vi "Calculate Normals.vi"(9 "Color Binding Mode":T1(ring), 10 "Vertex Array":cluster{"X":sgl, "Y":sgl, "Z":sgl}[](array[cluster]), 11 "Draw Mode":T2(ring)) -> (3 "Normal Array":cluster{"X":sgl, "Y":sgl, "Z":sgl}[](array[cluster]))   [LabVIEW 2023]
doc: "Calculates Normal values of the vertices."
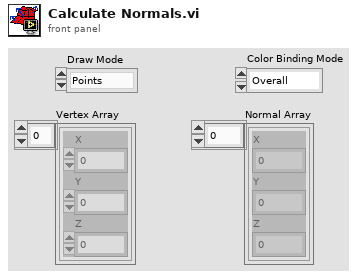
[diagram p1: front panel]
types:
  T1 = enum16{"Overall", "Per Primitive", "Per Vertex", "Binding Off"}
  T2 = enum16{"Points", "Lines", "Line Strip", "Line Loop", "Triangles", "Triangle Strip", "Triangle Fan", "Quads", "Quad Strip", "Polygon"}
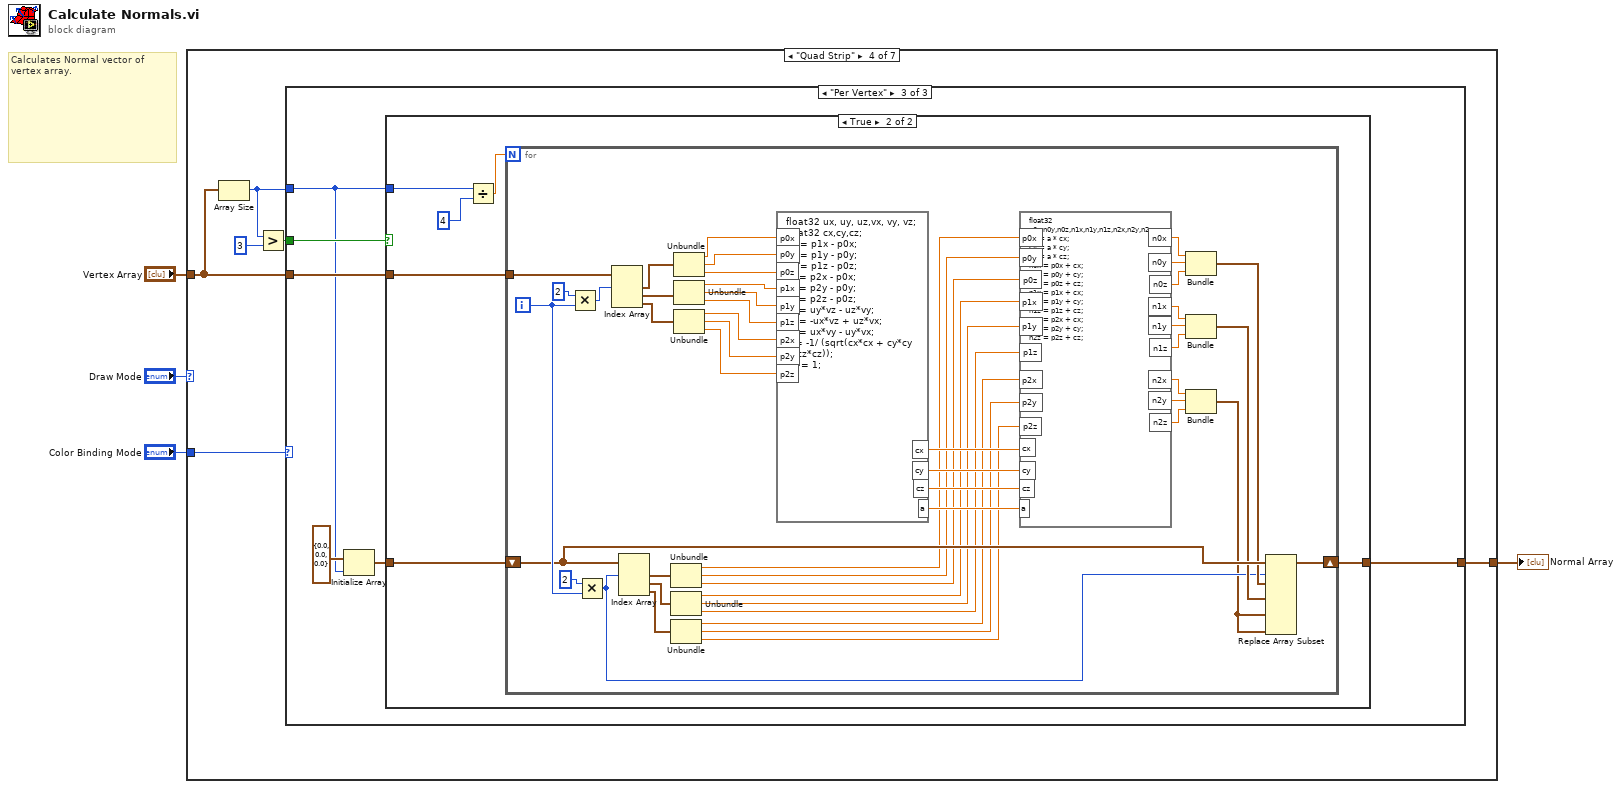
[diagram p0: block diagram]
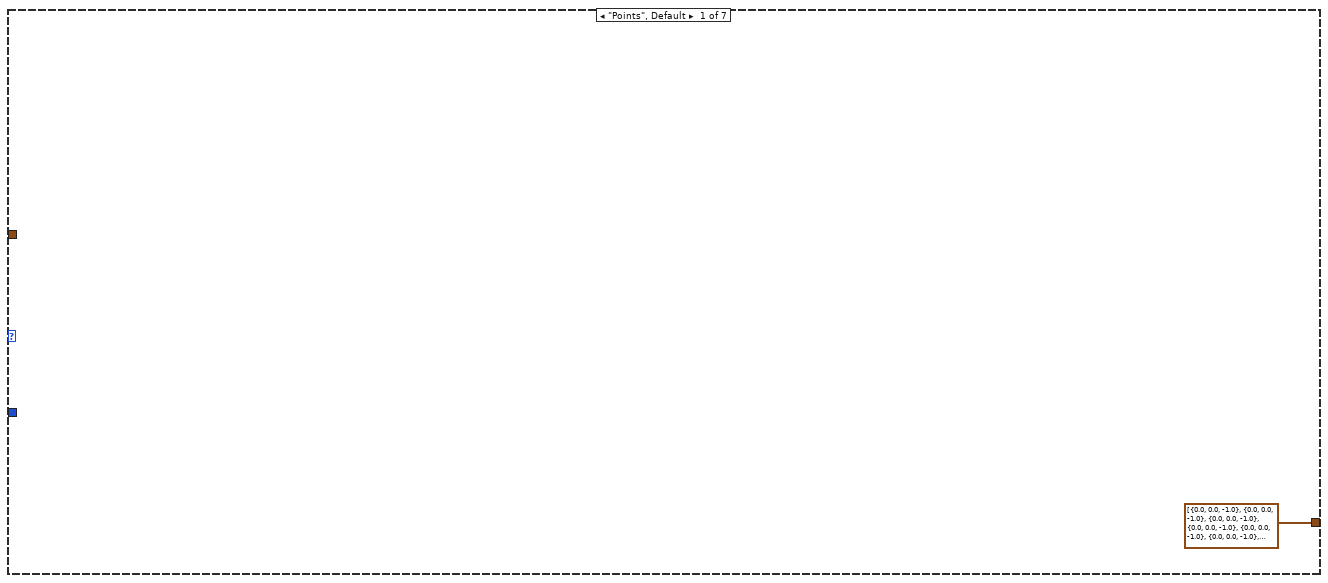
[diagram p2: hidden frame]
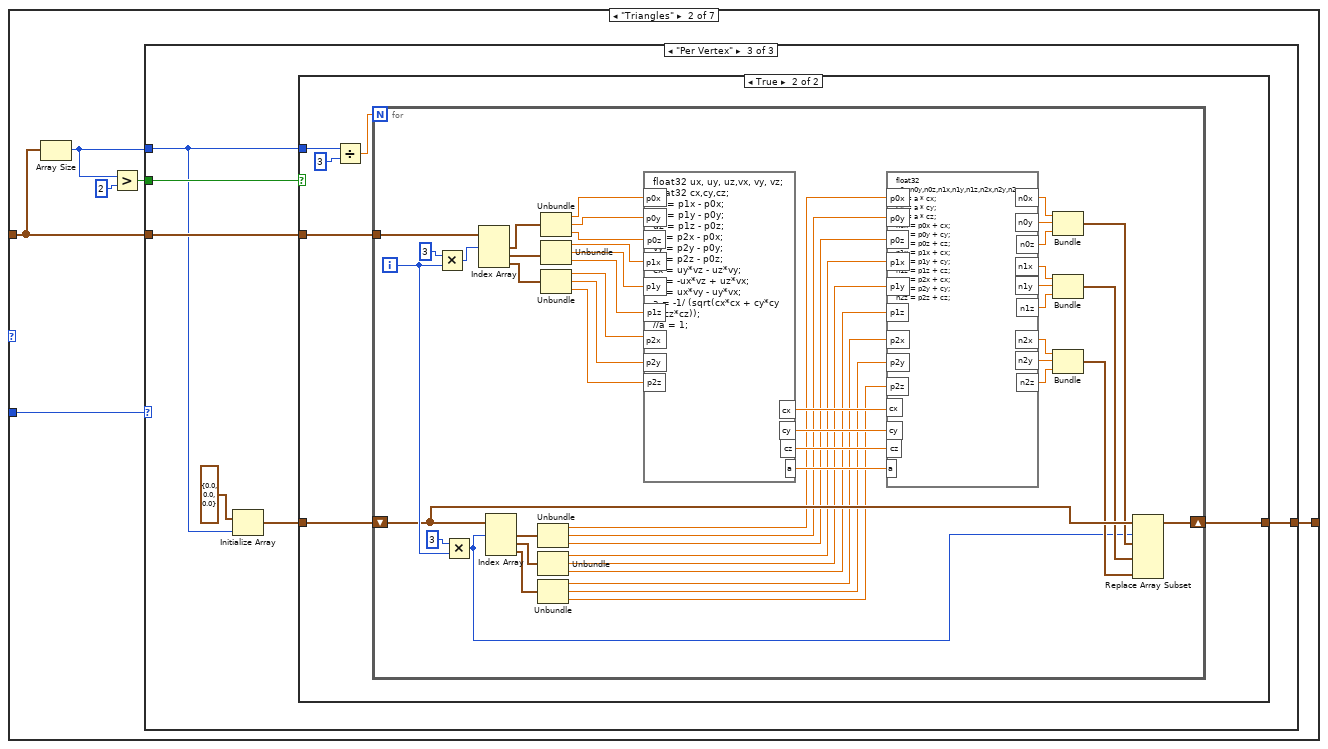
[diagram p3: hidden frame]
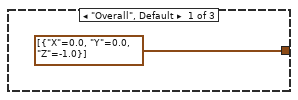
[diagram p4: hidden frame]
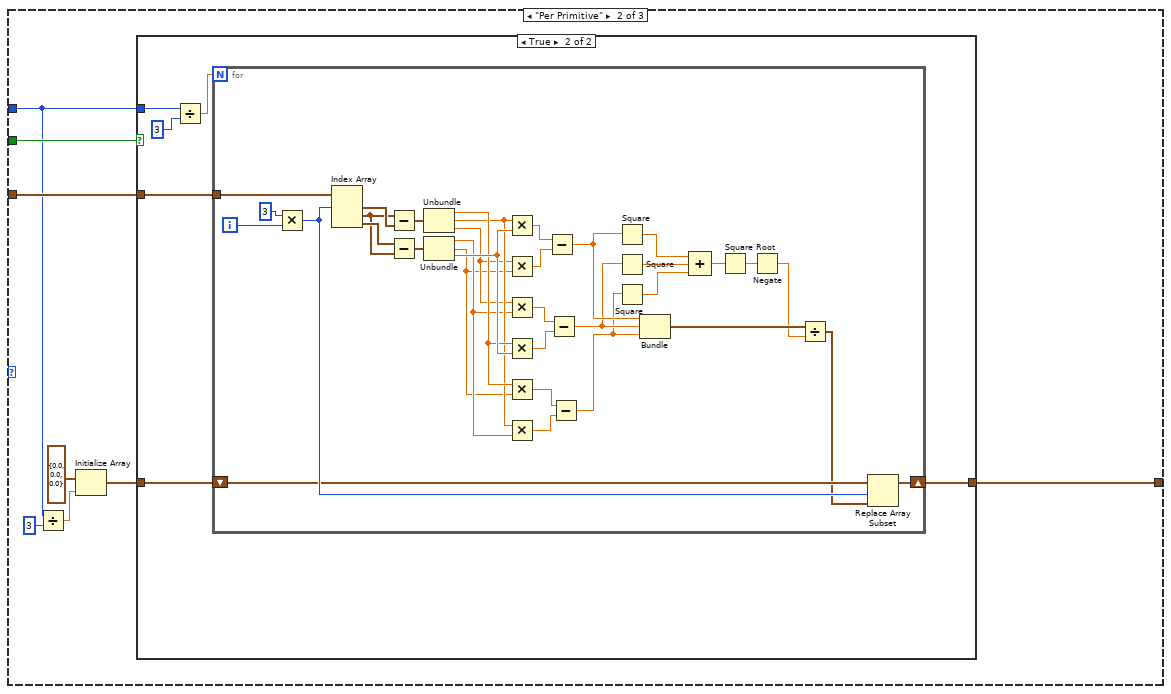
[diagram p5: hidden frame]
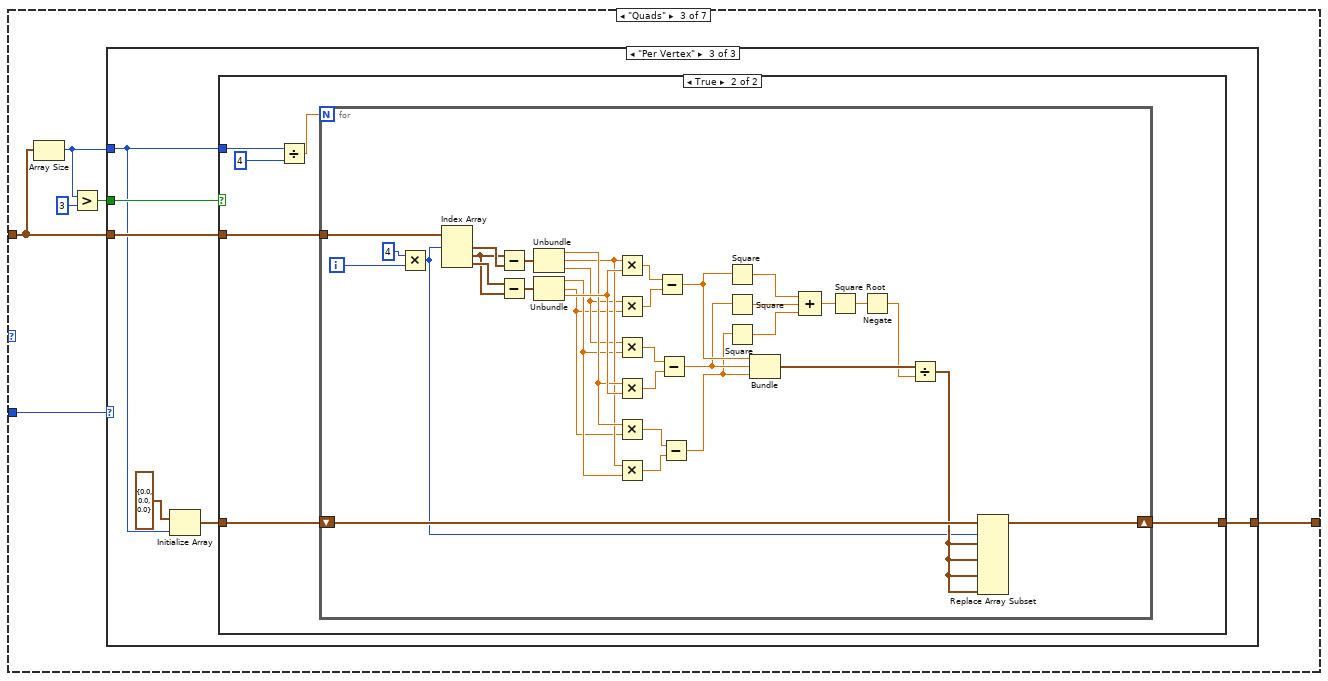
[diagram p8: hidden frame]
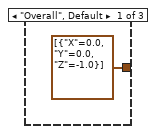
[diagram p9: hidden frame]
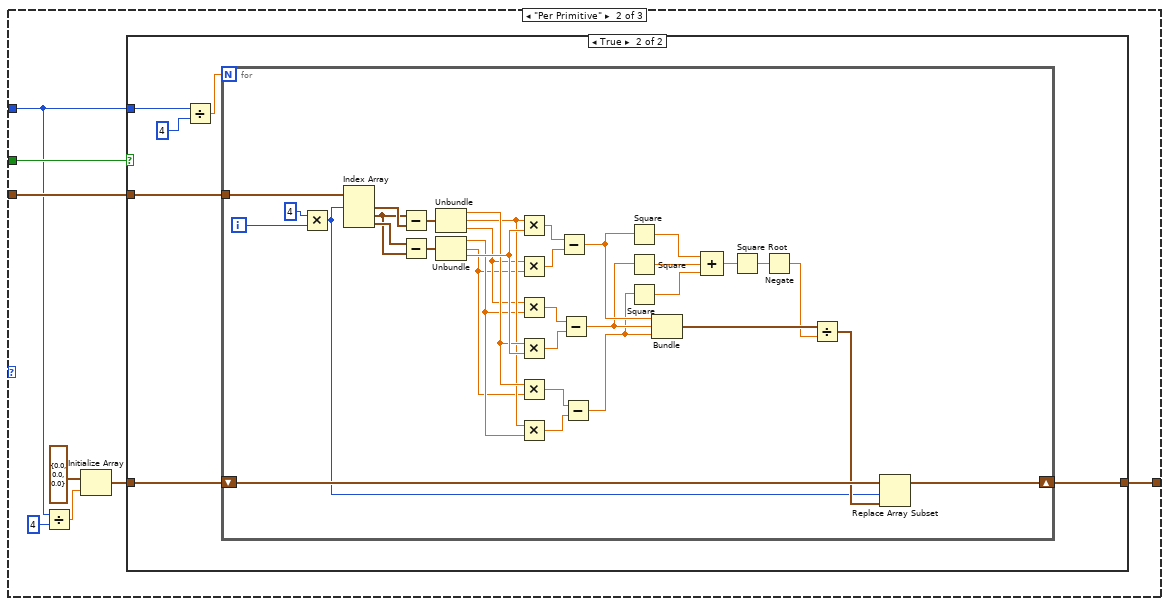
[diagram p10: hidden frame]
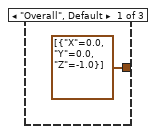
[diagram p13: hidden frame]
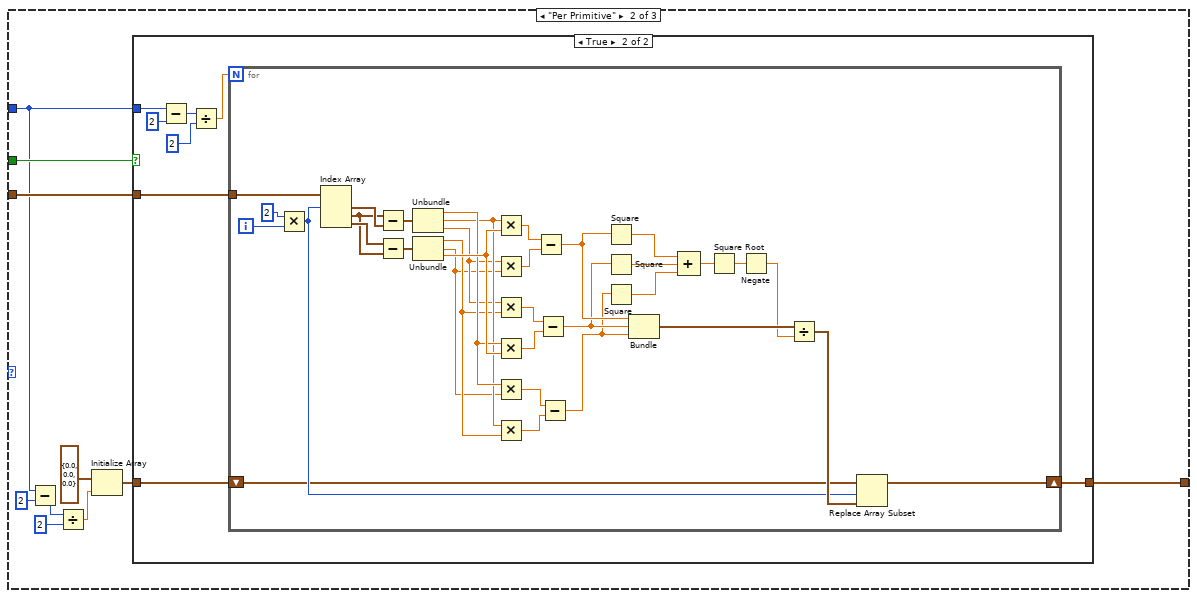
[diagram p14: hidden frame]
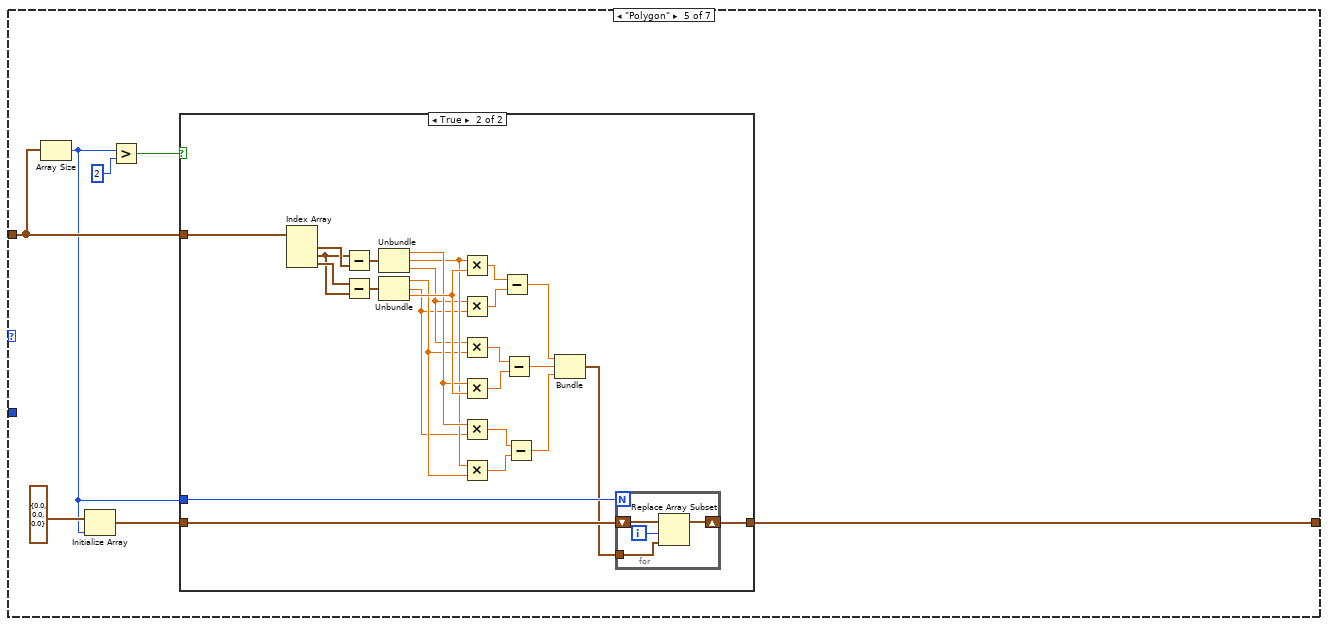
[diagram p17: hidden frame]
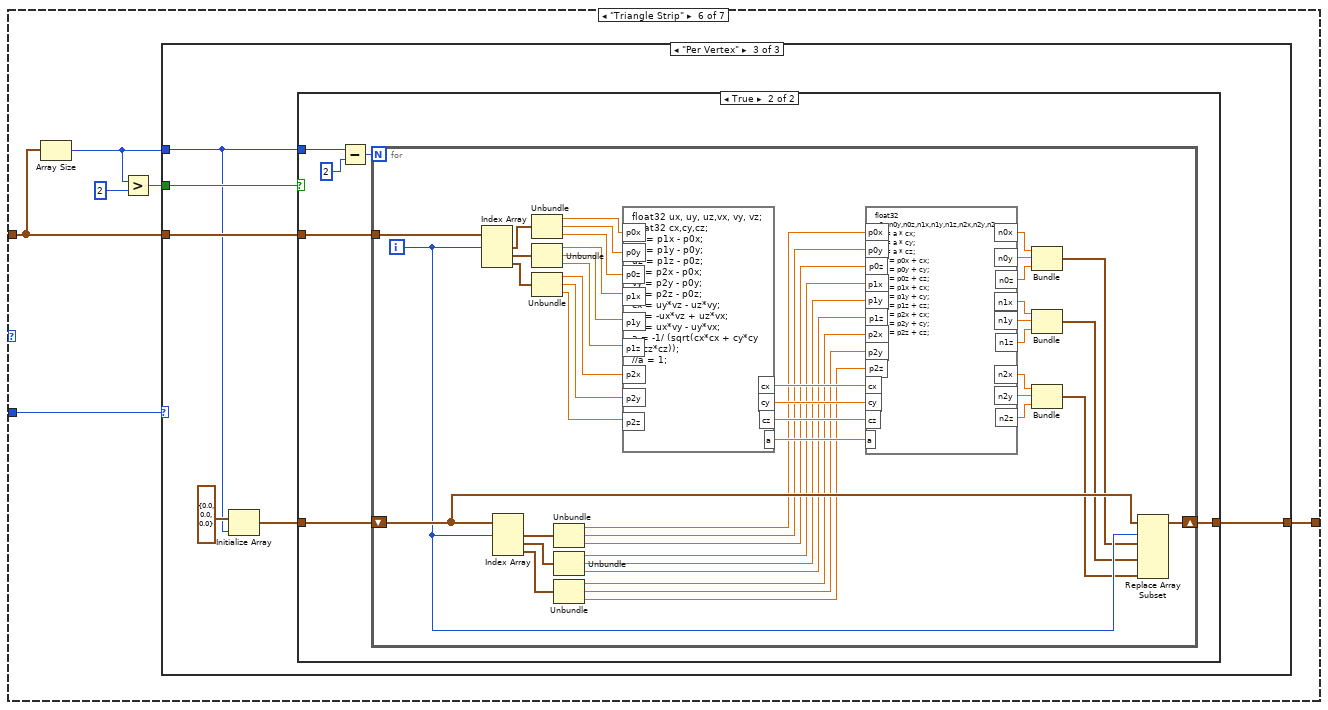
[diagram p19: hidden frame]
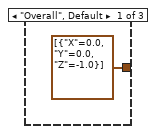
[diagram p20: hidden frame]
diagram:
  # "Calculates Normal vector of  vertex array."
  n1 = case shown="\"Quad Strip\"" "Draw Mode" {
    tunnel: "Vertex Array" -> [_ w11 w126 w227 w347 w382 w490]
    tunnel: [cluster{"X":sgl, "Y":sgl, "Z":sgl}[] [{"X"=0.0, "Y"=0.0, "Z"=-1.0}, {"X"=0.0, "Y"=0.0, "Z"=-1.0}, {"X"=0.0, "Y"=0.0, "Z"=-1.0}, {"X"=0.0, "Y"=0.0, "Z"=-1.0}, {"X"=0.0, "Y"=0.0, "Z"=-1.0}, {"X"=0.0, "Y"=0.0, "Z"=-1.0}, {"X"=0.0, "Y"=0.0, "Z"=-1.0}, {"X"=0.0, "Y"=0.0, "Z"=-1.0}, {"X"=0.0, "Y"=0.0, "Z"=-1.0}, {"X"=0.0, "Y"=0.0, "Z"=-1.0}] w10 w125 w226 w341 w381 w489] -> w2
    tunnel: "Color Binding Mode" -> [_ w7 w122 w222 _ w377 w485]
    frame "Points", Default {
    }
    frame "Triangles" {
      n2 = Array Size(array=w11) -> (size(s)=w6:i32)
      n3 = Greater?(x=w6, y=2) -> (0:w8:bool)
      n4 = case shown="\"Per Vertex\"" w7 {
        tunnel: w11 -> [_ w20 w66]
        tunnel: [cluster{"X":sgl, "Y":sgl, "Z":sgl}[] [{"X"=0.0, "Y"=0.0, "Z"=-1.0}] w19 w65] -> w10
        tunnel: w6 -> [_ w13 w61]
        tunnel: w8 -> [_ w18 w64]
        frame "Overall", Default {
        }
        frame "Per Primitive" {
          n5 = Divide(x=w13, y=3) -> (x/y=w15:dbl)
          n6 = Initialize Array(cluster{"X":sgl, "Y":sgl, "Z":sgl} {"X"=0.0, "Y"=0.0, "Z"=0.0} ("element"), w15) -> (w14:cluster{"X":sgl, "Y":sgl, "Z":sgl}[])
          n7 = case shown="True" w18 {
            tunnel: w20 -> [_ w26]
            tunnel: w14 -> [_ w23]
            tunnel: [_ w22] -> w19
            tunnel: w13 -> [_ w21]
            frame False {
            }
            frame True {
              n8 = Divide(x=w21, y=3) -> (x/y=w24:dbl)
              n9 = for {
                N: w24 -> [_]
                tunnel: w26 -> [w33]
                shift-right: [w29] -> w22
                shift-left: w23 -> [w31]
                i -> [w60]
                n10 = Multiply(x=3, y=w60) -> (x*y=w32:i32)
                n11 = Index Array(array=w33, index #1=w32) -> (element #1=w57:cluster{"X":sgl, "Y":sgl, "Z":sgl}, element #2=w56:cluster{"X":sgl, "Y":sgl, "Z":sgl}, element #3=w58:cluster{"X":sgl, "Y":sgl, "Z":sgl})  [unwired: 2 in]
                n12 = Subtract(x=w56, y=w57) -> (x-y=w54:cluster{"X":sgl, "Y":sgl, "Z":sgl})
                n13 = Subtract(x=w58, y=w56) -> (x-y=w55:cluster{"X":sgl, "Y":sgl, "Z":sgl})
                n14 = Unbundle(w54) -> ("X"=w52:sgl, "Y"=w51:sgl, "Z"=w50:sgl)
                n15 = Unbundle(w55) -> ("X"=w49:sgl, "Y"=w48:sgl, "Z"=w53:sgl)
                n16 = Multiply(x=w51, y=w53) -> (x*y=w47:sgl)
                n17 = Multiply(x=w50, y=w48) -> (x*y=w46:sgl)
                n18 = Multiply(x=w50, y=w49) -> (x*y=w44:sgl)
                n19 = Multiply(x=w52, y=w53) -> (x*y=w45:sgl)
                n20 = Multiply(x=w52, y=w48) -> (x*y=w42:sgl)
                n21 = Multiply(x=w51, y=w49) -> (x*y=w43:sgl)
                n22 = Subtract(x=w47, y=w46) -> (x-y=w39:sgl)
                n23 = Subtract(x=w44, y=w45) -> (x-y=w38:sgl)
                n24 = Subtract(x=w42, y=w43) -> (x-y=w37:sgl)
                n25 = Square(x=w39) -> (x^2=w28:sgl)
                n26 = Square(x=w38) -> (x^2=w27:sgl)
                n27 = Square(x=w37) -> (x^2=w41:sgl)
                n28 = Bundle(w39, w38, w37) -> (w36:cluster{sgl, sgl, sgl})  [unwired: 1 in]
                n29 = Compound Arithmetic op=ADD(w28, w27, w41) -> (w40:sgl)
                n30 = Square Root(x=w40) -> (sqrt(x)=w35:sgl)
                n31 = Negate(x=w35) -> (-x=w34:sgl)
                n32 = Divide(x=w36, y=w34) -> (x/y=w30:cluster{sgl, sgl, sgl})
                n33 = Replace Array Subset(array=w31, new element=w30, index=w32) -> (w29:cluster{"X":sgl, "Y":sgl, "Z":sgl}[])
              }
            }
          }
        }
        frame "Per Vertex" {
          n34 = Initialize Array(cluster{"X":sgl, "Y":sgl, "Z":sgl} {"X"=0.0, "Y"=0.0, "Z"=0.0} ("element"), w61) -> (w62:cluster{"X":sgl, "Y":sgl, "Z":sgl}[])
          n35 = case shown="True" w64 {
            tunnel: w66 -> [_ w72]
            tunnel: w62 -> [_ w69]
            tunnel: [_ w68] -> w65
            tunnel: w61 -> [_ w67]
            frame False {
            }
            frame True {
              n36 = Divide(x=w67, y=3) -> (x/y=w70:dbl)
              n37 = for {
                N: w70 -> [_]
                tunnel: w72 -> [w120]
                shift-right: [w117] -> w68
                shift-left: w69 -> [w118]
                i -> [w119]
                n38 = Multiply(x=3, y=w119) -> (x*y=w115:i32)
                n39 = Multiply(x=3, y=w119) -> (x*y=w73:i32)
                n40 = Index Array(array=w120, index #1=w115) -> (element #1=w98:cluster{"X":sgl, "Y":sgl, "Z":sgl}, element #2=w99:cluster{"X":sgl, "Y":sgl, "Z":sgl}, element #3=w100:cluster{"X":sgl, "Y":sgl, "Z":sgl})  [unwired: 2 in]
                n41 = Index Array(array=w118, index #1=w73) -> (element #1=w88:cluster{"X":sgl, "Y":sgl, "Z":sgl}, element #2=w87:cluster{"X":sgl, "Y":sgl, "Z":sgl}, element #3=w86:cluster{"X":sgl, "Y":sgl, "Z":sgl})  [unwired: 2 in]
                n42 = Unbundle(w88) -> ("X"=w85:sgl, "Y"=w84:sgl, "Z"=w83:sgl)
                n43 = Unbundle(w87) -> ("X"=w82:sgl, "Y"=w81:sgl, "Z"=w80:sgl)
                n44 = Unbundle(w86) -> ("X"=w79:sgl, "Y"=w78:sgl, "Z"=w77:sgl)
                n45 = Unbundle(w98) -> ("X"=w97:sgl, "Y"=w96:sgl, "Z"=w95:sgl)
                n46 = Unbundle(w99) -> ("X"=w94:sgl, "Y"=w93:sgl, "Z"=w92:sgl)
                n47 = Unbundle(w100) -> ("X"=w91:sgl, "Y"=w90:sgl, "Z"=w89:sgl)
                n48 = formula code="float32 ux, uy, uz,vx, vy, vz; \nfloat32 cx,cy,cz; \nux = p1x - p0x; \nuy = p1y - p0y; \nuz = p1z - p0z; \nvx = p2x - p0x; \nvy = p2y - p0y; \nvz = p2z - p0z; \ncx = uy*vz - uz*vy;\ncy = -ux*vz + uz*vx;\ncz = ux*vy - uy*vx;\na = -1/ (sqrt(cx*cx + cy*cy + cz*cz));\n//a = 1;"("p0x"=w97, "p0y"=w96, "p0z"=w95, "p1x"=w94, "p1y"=w93, "p1z"=w92, "p2x"=w91, "p2y"=w90, "p2z"=w89) -> ("cx"=w104:sgl, "cy"=w103:sgl, "cz"=w102:sgl, "a"=w105:dbl)
                n49 = formula code="float32 n0x,n0y,n0z,n1x,n1y,n1z,n2x,n2y,n2z;\ncx = a * cx; \ncy = a * cy; \ncz = a * cz; \nn0x = p0x + cx; \nn0y = p0y + cy;\nn0z = p0z + cz;\nn1x = p1x + cx; \nn1y = p1y + cy;\nn1z = p1z + cz;\nn2x = p2x + cx; \nn2y = p2y + cy;\nn2z = p2z + cz;"("p0x"=w85, "p0y"=w84, "p0z"=w83, "p1x"=w82, "p1y"=w81, "p1z"=w80, "p2x"=w79, "p2y"=w78, "p2z"=w77, "cx"=w104, "cy"=w103, "cz"=w102, "a"=w105) -> ("n0x"=w114:sgl, "n0y"=w113:sgl, "n0z"=w112:sgl, "n1x"=w111:sgl, "n1y"=w110:sgl, "n1z"=w109:sgl, "n2x"=w108:sgl, "n2y"=w107:sgl, "n2z"=w106:sgl)
                n50 = Bundle(w114, w113, w112) -> (w76:cluster{sgl, sgl, sgl})  [unwired: 1 in]
                n51 = Bundle(w111, w110, w109) -> (w75:cluster{sgl, sgl, sgl})  [unwired: 1 in]
                n52 = Bundle(w108, w107, w106) -> (w74:cluster{sgl, sgl, sgl})  [unwired: 1 in]
                n53 = Replace Array Subset(array=w118, new element #1=w76, index #1=w73, new element #2=w75, new element #3=w74) -> (w117:cluster{"X":sgl, "Y":sgl, "Z":sgl}[])  [unwired: 2 in]
              }
            }
          }
        }
      }
    }
    frame "Quads" {
      n54 = Array Size(array=w126) -> (size(s)=w121:i32)
      n55 = Greater?(x=w121, y=3) -> (0:w123:bool)
      n56 = case shown="\"Per Vertex\"" w122 {
        tunnel: w126 -> [_ w135 w181]
        tunnel: [cluster{"X":sgl, "Y":sgl, "Z":sgl}[] [{"X"=0.0, "Y"=0.0, "Z"=-1.0}] w134 w180] -> w125
        tunnel: w121 -> [_ w128 w177]
        tunnel: w123 -> [_ w133 w179]
        frame "Overall", Default {
        }
        frame "Per Primitive" {
          n57 = Divide(x=w128, y=4) -> (x/y=w130:dbl)
          n58 = Initialize Array(cluster{"X":sgl, "Y":sgl, "Z":sgl} {"X"=0.0, "Y"=0.0, "Z"=0.0} ("element"), w130) -> (w129:cluster{"X":sgl, "Y":sgl, "Z":sgl}[])
          n59 = case shown="True" w133 {
            tunnel: w135 -> [_ w139]
            tunnel: w129 -> [_ w137]
            tunnel: [_ w136] -> w134
            tunnel: w128 -> [_ w140]
            frame False {
            }
            frame True {
              n60 = Divide(x=w140, y=4) -> (x/y=w138:dbl)
              n61 = for {
                N: w138 -> [_]
                tunnel: w139 -> [w175]
                shift-right: [w172] -> w136
                shift-left: w137 -> [w173]
                i -> [w174]
                n62 = Multiply(x=4, y=w174) -> (x*y=w145:i32)
                n63 = Index Array(array=w175, index #1=w145) -> (element #1=w169:cluster{"X":sgl, "Y":sgl, "Z":sgl}, element #2=w168:cluster{"X":sgl, "Y":sgl, "Z":sgl}, element #3=w170:cluster{"X":sgl, "Y":sgl, "Z":sgl})  [unwired: 2 in]
                n64 = Subtract(x=w168, y=w169) -> (x-y=w166:cluster{"X":sgl, "Y":sgl, "Z":sgl})
                n65 = Subtract(x=w170, y=w168) -> (x-y=w167:cluster{"X":sgl, "Y":sgl, "Z":sgl})
                n66 = Unbundle(w166) -> ("X"=w164:sgl, "Y"=w163:sgl, "Z"=w162:sgl)
                n67 = Unbundle(w167) -> ("X"=w161:sgl, "Y"=w160:sgl, "Z"=w165:sgl)
                n68 = Multiply(x=w163, y=w165) -> (x*y=w159:sgl)
                n69 = Multiply(x=w162, y=w160) -> (x*y=w158:sgl)
                n70 = Multiply(x=w162, y=w161) -> (x*y=w156:sgl)
                n71 = Multiply(x=w164, y=w165) -> (x*y=w157:sgl)
                n72 = Multiply(x=w164, y=w160) -> (x*y=w154:sgl)
                n73 = Multiply(x=w163, y=w161) -> (x*y=w155:sgl)
                n74 = Subtract(x=w159, y=w158) -> (x-y=w151:sgl)
                n75 = Subtract(x=w156, y=w157) -> (x-y=w150:sgl)
                n76 = Subtract(x=w154, y=w155) -> (x-y=w149:sgl)
                n77 = Square(x=w151) -> (x^2=w143:sgl)
                n78 = Square(x=w150) -> (x^2=w142:sgl)
                n79 = Square(x=w149) -> (x^2=w153:sgl)
                n80 = Bundle(w151, w150, w149) -> (w148:cluster{sgl, sgl, sgl})  [unwired: 1 in]
                n81 = Compound Arithmetic op=ADD(w143, w142, w153) -> (w152:sgl)
                n82 = Square Root(x=w152) -> (sqrt(x)=w147:sgl)
                n83 = Negate(x=w147) -> (-x=w144:sgl)
                n84 = Divide(x=w148, y=w144) -> (x/y=w146:cluster{sgl, sgl, sgl})
                n85 = Replace Array Subset(array=w173, new element=w146, index=w145) -> (w172:cluster{"X":sgl, "Y":sgl, "Z":sgl}[])
              }
            }
          }
        }
        frame "Per Vertex" {
          n86 = Initialize Array(cluster{"X":sgl, "Y":sgl, "Z":sgl} {"X"=0.0, "Y"=0.0, "Z"=0.0} ("element"), w177) -> (w176:cluster{"X":sgl, "Y":sgl, "Z":sgl}[])
          n87 = case shown="True" w179 {
            tunnel: w181 -> [_ w185]
            tunnel: w176 -> [_ w183]
            tunnel: [_ w182] -> w180
            tunnel: w177 -> [_ w186]
            frame False {
            }
            frame True {
              n88 = Divide(x=w186, y=4) -> (x/y=w184:dbl)
              n89 = for {
                N: w184 -> [_]
                tunnel: w185 -> [w221]
                shift-right: [w218] -> w182
                shift-left: w183 -> [w219]
                i -> [w220]
                n90 = Multiply(x=4, y=w220) -> (x*y=w191:i32)
                n91 = Index Array(array=w221, index #1=w191) -> (element #1=w215:cluster{"X":sgl, "Y":sgl, "Z":sgl}, element #2=w214:cluster{"X":sgl, "Y":sgl, "Z":sgl}, element #3=w216:cluster{"X":sgl, "Y":sgl, "Z":sgl})  [unwired: 2 in]
                n92 = Subtract(x=w214, y=w215) -> (x-y=w212:cluster{"X":sgl, "Y":sgl, "Z":sgl})
                n93 = Subtract(x=w216, y=w214) -> (x-y=w213:cluster{"X":sgl, "Y":sgl, "Z":sgl})
                n94 = Unbundle(w212) -> ("X"=w210:sgl, "Y"=w209:sgl, "Z"=w208:sgl)
                n95 = Unbundle(w213) -> ("X"=w207:sgl, "Y"=w206:sgl, "Z"=w211:sgl)
                n96 = Multiply(x=w209, y=w211) -> (x*y=w205:sgl)
                n97 = Multiply(x=w208, y=w206) -> (x*y=w204:sgl)
                n98 = Multiply(x=w208, y=w207) -> (x*y=w202:sgl)
                n99 = Multiply(x=w210, y=w211) -> (x*y=w203:sgl)
                n100 = Multiply(x=w210, y=w206) -> (x*y=w200:sgl)
                n101 = Multiply(x=w209, y=w207) -> (x*y=w201:sgl)
                n102 = Subtract(x=w205, y=w204) -> (x-y=w197:sgl)
                n103 = Subtract(x=w202, y=w203) -> (x-y=w196:sgl)
                n104 = Subtract(x=w200, y=w201) -> (x-y=w195:sgl)
                n105 = Square(x=w197) -> (x^2=w189:sgl)
                n106 = Square(x=w196) -> (x^2=w188:sgl)
                n107 = Square(x=w195) -> (x^2=w199:sgl)
                n108 = Bundle(w197, w196, w195) -> (w194:cluster{sgl, sgl, sgl})  [unwired: 1 in]
                n109 = Compound Arithmetic op=ADD(w189, w188, w199) -> (w198:sgl)
                n110 = Square Root(x=w198) -> (sqrt(x)=w193:sgl)
                n111 = Negate(x=w193) -> (-x=w190:sgl)
                n112 = Divide(x=w194, y=w190) -> (x/y=w192:cluster{sgl, sgl, sgl})
                n113 = Replace Array Subset(array=w219, new element #1=w192, index #1=w191, new element #2=w192, new element #3=w192, new element #4=w192) -> (w218:cluster{"X":sgl, "Y":sgl, "Z":sgl}[])  [unwired: 3 in]
              }
            }
          }
        }
      }
    }
    frame "Quad Strip" {
      n114 = Array Size(array=w227) -> (size(s)=w225:i32)
      n115 = Greater?(x=w225, y=3) -> (0:w223:bool)
      n116 = case shown="\"Per Vertex\"" w222 {
        tunnel: w227 -> [_ w238 w286]
        tunnel: [cluster{"X":sgl, "Y":sgl, "Z":sgl}[] [{"X"=0.0, "Y"=0.0, "Z"=-1.0}] w237 w285] -> w226
        tunnel: w225 -> [_ w230 w281]
        tunnel: w223 -> [_ w236 w284]
        frame "Overall", Default {
        }
        frame "Per Primitive" {
          n117 = Subtract(x=w230, y=2) -> (x-y=w229:i32)
          n118 = Divide(x=w229, y=2) -> (x/y=w232:dbl)
          n119 = Initialize Array(cluster{"X":sgl, "Y":sgl, "Z":sgl} {"X"=0.0, "Y"=0.0, "Z"=0.0} ("element"), w232) -> (w234:cluster{"X":sgl, "Y":sgl, "Z":sgl}[])
          n120 = case shown="True" w236 {
            tunnel: w238 -> [_ w245]
            tunnel: w234 -> [_ w243]
            tunnel: [_ w242] -> w237
            tunnel: w230 -> [_ w240]
            frame False {
            }
            frame True {
              n121 = Subtract(x=w240, y=2) -> (x-y=w239:i32)
              n122 = Divide(x=w239, y=2) -> (x/y=w244:dbl)
              n123 = for {
                N: w244 -> [_]
                tunnel: w245 -> [w252]
                shift-right: [w249] -> w242
                shift-left: w243 -> [w250]
                i -> [w251]
                n124 = Multiply(x=2, y=w251) -> (x*y=w254:i32)
                n125 = Index Array(array=w252, index #1=w254) -> (element #1=w278:cluster{"X":sgl, "Y":sgl, "Z":sgl}, element #2=w277:cluster{"X":sgl, "Y":sgl, "Z":sgl}, element #3=w279:cluster{"X":sgl, "Y":sgl, "Z":sgl})  [unwired: 2 in]
                n126 = Subtract(x=w277, y=w278) -> (x-y=w275:cluster{"X":sgl, "Y":sgl, "Z":sgl})
                n127 = Subtract(x=w279, y=w277) -> (x-y=w276:cluster{"X":sgl, "Y":sgl, "Z":sgl})
                n128 = Unbundle(w275) -> ("X"=w273:sgl, "Y"=w272:sgl, "Z"=w271:sgl)
                n129 = Unbundle(w276) -> ("X"=w270:sgl, "Y"=w269:sgl, "Z"=w274:sgl)
                n130 = Multiply(x=w272, y=w274) -> (x*y=w268:sgl)
                n131 = Multiply(x=w271, y=w269) -> (x*y=w267:sgl)
                n132 = Multiply(x=w271, y=w270) -> (x*y=w265:sgl)
                n133 = Multiply(x=w273, y=w274) -> (x*y=w266:sgl)
                n134 = Multiply(x=w273, y=w269) -> (x*y=w263:sgl)
                n135 = Multiply(x=w272, y=w270) -> (x*y=w264:sgl)
                n136 = Subtract(x=w268, y=w267) -> (x-y=w260:sgl)
                n137 = Subtract(x=w265, y=w266) -> (x-y=w259:sgl)
                n138 = Subtract(x=w263, y=w264) -> (x-y=w258:sgl)
                n139 = Square(x=w260) -> (x^2=w247:sgl)
                n140 = Square(x=w259) -> (x^2=w248:sgl)
                n141 = Square(x=w258) -> (x^2=w262:sgl)
                n142 = Bundle(w260, w259, w258) -> (w257:cluster{sgl, sgl, sgl})  [unwired: 1 in]
                n143 = Compound Arithmetic op=ADD(w247, w248, w262) -> (w261:sgl)
                n144 = Square Root(x=w261) -> (sqrt(x)=w256:sgl)
                n145 = Negate(x=w256) -> (-x=w253:sgl)
                n146 = Divide(x=w257, y=w253) -> (x/y=w255:cluster{sgl, sgl, sgl})
                n147 = Replace Array Subset(array=w250, new element=w255, index=w254) -> (w249:cluster{"X":sgl, "Y":sgl, "Z":sgl}[])
              }
            }
          }
        }
        frame "Per Vertex" {
          n148 = Initialize Array(cluster{"X":sgl, "Y":sgl, "Z":sgl} {"X"=0.0, "Y"=0.0, "Z"=0.0} ("element"), w281) -> (w282:cluster{"X":sgl, "Y":sgl, "Z":sgl}[])
          n149 = case shown="True" w284 {
            tunnel: w286 -> [_ w290]
            tunnel: w282 -> [_ w288]
            tunnel: [_ w287] -> w285
            tunnel: w281 -> [_ w291]
            frame False {
            }
            frame True {
              n150 = Divide(x=w291, y=4) -> (x/y=w289:dbl)
              n151 = for {
                N: w289 -> [_]
                tunnel: w290 -> [w340]
                shift-right: [w337] -> w287
                shift-left: w288 -> [w338]
                i -> [w339]
                n152 = Multiply(x=2, y=w339) -> (x*y=w335:i32)
                n153 = Multiply(x=2, y=w339) -> (x*y=w294:i32)
                n154 = Index Array(array=w340, index #1=w335) -> (element #1=w318:cluster{"X":sgl, "Y":sgl, "Z":sgl}, element #2=w319:cluster{"X":sgl, "Y":sgl, "Z":sgl}, element #3=w320:cluster{"X":sgl, "Y":sgl, "Z":sgl})  [unwired: 2 in]
                n155 = Index Array(array=w338, index #1=w294) -> (element #1=w308:cluster{"X":sgl, "Y":sgl, "Z":sgl}, element #2=w307:cluster{"X":sgl, "Y":sgl, "Z":sgl}, element #3=w306:cluster{"X":sgl, "Y":sgl, "Z":sgl})  [unwired: 2 in]
                n156 = Unbundle(w308) -> ("X"=w305:sgl, "Y"=w304:sgl, "Z"=w303:sgl)
                n157 = Unbundle(w307) -> ("X"=w302:sgl, "Y"=w301:sgl, "Z"=w300:sgl)
                n158 = Unbundle(w306) -> ("X"=w299:sgl, "Y"=w298:sgl, "Z"=w297:sgl)
                n159 = Unbundle(w318) -> ("X"=w317:sgl, "Y"=w316:sgl, "Z"=w315:sgl)
                n160 = Unbundle(w319) -> ("X"=w314:sgl, "Y"=w313:sgl, "Z"=w312:sgl)
                n161 = Unbundle(w320) -> ("X"=w311:sgl, "Y"=w310:sgl, "Z"=w309:sgl)
                n162 = formula code="float32 ux, uy, uz,vx, vy, vz; \nfloat32 cx,cy,cz; \nux = p1x - p0x; \nuy = p1y - p0y; \nuz = p1z - p0z; \nvx = p2x - p0x; \nvy = p2y - p0y; \nvz = p2z - p0z; \ncx = uy*vz - uz*vy;\ncy = -ux*vz + uz*vx;\ncz = ux*vy - uy*vx;\na = -1/ (sqrt(cx*cx + cy*cy + cz*cz));\n//a = 1;"("p0x"=w317, "p0y"=w316, "p0z"=w315, "p1x"=w314, "p1y"=w313, "p1z"=w312, "p2x"=w311, "p2y"=w310, "p2z"=w309) -> ("cx"=w324:sgl, "cy"=w323:sgl, "cz"=w322:sgl, "a"=w325:dbl)
                n163 = formula code="float32 n0x,n0y,n0z,n1x,n1y,n1z,n2x,n2y,n2z;\ncx = a * cx; \ncy = a * cy; \ncz = a * cz; \nn0x = p0x + cx; \nn0y = p0y + cy;\nn0z = p0z + cz;\nn1x = p1x + cx; \nn1y = p1y + cy;\nn1z = p1z + cz;\nn2x = p2x + cx; \nn2y = p2y + cy;\nn2z = p2z + cz;"("p0x"=w305, "p0y"=w304, "p0z"=w303, "p1x"=w302, "p1y"=w301, "p1z"=w300, "p2x"=w299, "p2y"=w298, "p2z"=w297, "cx"=w324, "cy"=w323, "cz"=w322, "a"=w325) -> ("n0x"=w334:sgl, "n0y"=w333:sgl, "n0z"=w332:sgl, "n1x"=w331:sgl, "n1y"=w330:sgl, "n1z"=w329:sgl, "n2x"=w328:sgl, "n2y"=w327:sgl, "n2z"=w326:sgl)
                n164 = Bundle(w334, w333, w332) -> (w296:cluster{sgl, sgl, sgl})  [unwired: 1 in]
                n165 = Bundle(w331, w330, w329) -> (w295:cluster{sgl, sgl, sgl})  [unwired: 1 in]
                n166 = Bundle(w328, w327, w326) -> (w293:cluster{sgl, sgl, sgl})  [unwired: 1 in]
                n167 = Replace Array Subset(array=w338, new element #1=w296, index #1=w294, new element #2=w295, new element #3=w293, new element #4=w293) -> (w337:cluster{"X":sgl, "Y":sgl, "Z":sgl}[])  [unwired: 3 in]
              }
            }
          }
        }
      }
    }
    frame "Polygon" {
      n168 = Array Size(array=w347) -> (size(s)=w342:i32)
      n169 = Initialize Array(cluster{"X":sgl, "Y":sgl, "Z":sgl} {"X"=0.0, "Y"=0.0, "Z"=0.0} ("element"), w342) -> (w345:cluster{"X":sgl, "Y":sgl, "Z":sgl}[])
      n170 = Greater?(x=w342, y=2) -> (0:w343:bool)
      n171 = case shown="True" w343 {
        tunnel: w347 -> [_ w372]
        tunnel: w345 -> [_ w350]
        tunnel: w342 -> [_ w351]
        tunnel: [_ w348] -> w341
        frame False {
        }
        frame True {
          n172 = Index Array(array=w372) -> (element #1=w370:cluster{"X":sgl, "Y":sgl, "Z":sgl}, element #2=w369:cluster{"X":sgl, "Y":sgl, "Z":sgl}, element #3=w371:cluster{"X":sgl, "Y":sgl, "Z":sgl})  [unwired: 3 in]
          n173 = Subtract(x=w369, y=w370) -> (x-y=w367:cluster{"X":sgl, "Y":sgl, "Z":sgl})
          n174 = Subtract(x=w371, y=w369) -> (x-y=w368:cluster{"X":sgl, "Y":sgl, "Z":sgl})
          n175 = Unbundle(w367) -> ("X"=w365:sgl, "Y"=w364:sgl, "Z"=w363:sgl)
          n176 = Unbundle(w368) -> ("X"=w362:sgl, "Y"=w361:sgl, "Z"=w366:sgl)
          n177 = Multiply(x=w364, y=w366) -> (x*y=w360:sgl)
          n178 = Multiply(x=w363, y=w361) -> (x*y=w359:sgl)
          n179 = Multiply(x=w363, y=w362) -> (x*y=w357:sgl)
          n180 = Multiply(x=w365, y=w366) -> (x*y=w358:sgl)
          n181 = Multiply(x=w365, y=w361) -> (x*y=w355:sgl)
          n182 = Multiply(x=w364, y=w362) -> (x*y=w356:sgl)
          n183 = Subtract(x=w360, y=w359) -> (x-y=w353:sgl)
          n184 = Subtract(x=w357, y=w358) -> (x-y=w354:sgl)
          n185 = Subtract(x=w355, y=w356) -> (x-y=w352:sgl)
          n186 = Bundle(w353, w354, w352) -> (w349:cluster{sgl, sgl, sgl})  [unwired: 1 in]
          n187 = for {
            N: w351 -> [_]
            shift-right: [w373] -> w348
            shift-left: w350 -> [w376]
            tunnel: w349 -> [w374]
            i -> [w375]
            n188 = Replace Array Subset(array=w376, new element=w374, index=w375) -> (w373:cluster{"X":sgl, "Y":sgl, "Z":sgl}[])
          }
        }
      }
    }
    frame "Triangle Strip" {
      n189 = Array Size(array=w382) -> (size(s)=w378:i32)
      n190 = Greater?(x=w378, y=2) -> (0:w379:bool)
      n191 = case shown="\"Per Vertex\"" w377 {
        tunnel: w382 -> [_ w391 w434]
        tunnel: [cluster{"X":sgl, "Y":sgl, "Z":sgl}[] [{"X"=0.0, "Y"=0.0, "Z"=-1.0}] w390 w433] -> w381
        tunnel: w379 -> [_ w389 w432]
        tunnel: w378 -> [_ w384 w429]
        frame "Overall", Default {
        }
        frame "Per Primitive" {
          n192 = Subtract(x=w384, y=2) -> (x-y=w385:i32)
          n193 = Initialize Array(cluster{"X":sgl, "Y":sgl, "Z":sgl} {"X"=0.0, "Y"=0.0, "Z"=0.0} ("element"), w385) -> (w387:cluster{"X":sgl, "Y":sgl, "Z":sgl}[])
          n194 = case shown="True" w389 {
            tunnel: w391 -> [_ w397]
            tunnel: w387 -> [_ w396]
            tunnel: [_ w395] -> w390
            tunnel: w384 -> [_ w394]
            frame False {
            }
            frame True {
              n195 = Subtract(x=w394, y=2) -> (x-y=w393:i32)
              n196 = for {
                N: w393 -> [_]
                tunnel: w397 -> [w404]
                shift-right: [w402] -> w395
                shift-left: w396 -> [w403]
                i -> [w401]
                n197 = Index Array(array=w404, index #1=w401) -> (element #1=w427:cluster{"X":sgl, "Y":sgl, "Z":sgl}, element #2=w426:cluster{"X":sgl, "Y":sgl, "Z":sgl}, element #3=w428:cluster{"X":sgl, "Y":sgl, "Z":sgl})  [unwired: 2 in]
                n198 = Subtract(x=w426, y=w427) -> (x-y=w424:cluster{"X":sgl, "Y":sgl, "Z":sgl})
                n199 = Subtract(x=w428, y=w426) -> (x-y=w425:cluster{"X":sgl, "Y":sgl, "Z":sgl})
                n200 = Unbundle(w424) -> ("X"=w422:sgl, "Y"=w421:sgl, "Z"=w420:sgl)
                n201 = Unbundle(w425) -> ("X"=w419:sgl, "Y"=w418:sgl, "Z"=w423:sgl)
                n202 = Multiply(x=w421, y=w423) -> (x*y=w417:sgl)
                n203 = Multiply(x=w420, y=w418) -> (x*y=w416:sgl)
                n204 = Multiply(x=w420, y=w419) -> (x*y=w414:sgl)
                n205 = Multiply(x=w422, y=w423) -> (x*y=w415:sgl)
                n206 = Multiply(x=w422, y=w418) -> (x*y=w412:sgl)
                n207 = Multiply(x=w421, y=w419) -> (x*y=w413:sgl)
                n208 = Subtract(x=w417, y=w416) -> (x-y=w409:sgl)
                n209 = Subtract(x=w414, y=w415) -> (x-y=w408:sgl)
                n210 = Subtract(x=w412, y=w413) -> (x-y=w407:sgl)
                n211 = Square(x=w409) -> (x^2=w399:sgl)
                n212 = Square(x=w408) -> (x^2=w398:sgl)
                n213 = Square(x=w407) -> (x^2=w411:sgl)
                n214 = Bundle(w409, w408, w407) -> (w406:cluster{sgl, sgl, sgl})  [unwired: 1 in]
                n215 = Compound Arithmetic op=ADD(w399, w398, w411) -> (w410:sgl)
                n216 = Square Root(x=w410) -> (sqrt(x)=w400:sgl)
                n217 = Divide(x=w406, y=w400) -> (x/y=w405:cluster{sgl, sgl, sgl})
                n218 = Replace Array Subset(array=w403, new element=w405, index=w401) -> (w402:cluster{"X":sgl, "Y":sgl, "Z":sgl}[])
              }
            }
          }
        }
        frame "Per Vertex" {
          n219 = Initialize Array(cluster{"X":sgl, "Y":sgl, "Z":sgl} {"X"=0.0, "Y"=0.0, "Z"=0.0} ("element"), w429) -> (w430:cluster{"X":sgl, "Y":sgl, "Z":sgl}[])
          n220 = case shown="True" w432 {
            tunnel: w434 -> [_ w440]
            tunnel: w430 -> [_ w439]
            tunnel: [_ w438] -> w433
            tunnel: w429 -> [_ w437]
            frame False {
            }
            frame True {
              n221 = Subtract(x=w437, y=2) -> (x-y=w436:i32)
              n222 = for {
                N: w436 -> [_]
                tunnel: w440 -> [w484]
                shift-right: [w482] -> w438
                shift-left: w439 -> [w483]
                i -> [w481]
                n223 = Index Array(array=w484, index #1=w481) -> (element #1=w466:cluster{"X":sgl, "Y":sgl, "Z":sgl}, element #2=w467:cluster{"X":sgl, "Y":sgl, "Z":sgl}, element #3=w465:cluster{"X":sgl, "Y":sgl, "Z":sgl})  [unwired: 2 in]
                n224 = Index Array(array=w483, index #1=w481) -> (element #1=w464:cluster{"X":sgl, "Y":sgl, "Z":sgl}, element #2=w463:cluster{"X":sgl, "Y":sgl, "Z":sgl}, element #3=w462:cluster{"X":sgl, "Y":sgl, "Z":sgl})  [unwired: 2 in]
                n225 = Unbundle(w466) -> ("X"=w461:sgl, "Y"=w460:sgl, "Z"=w459:sgl)
                n226 = Unbundle(w467) -> ("X"=w458:sgl, "Y"=w457:sgl, "Z"=w456:sgl)
                n227 = Unbundle(w465) -> ("X"=w455:sgl, "Y"=w454:sgl, "Z"=w453:sgl)
                n228 = Unbundle(w464) -> ("X"=w452:sgl, "Y"=w451:sgl, "Z"=w450:sgl)
                n229 = Unbundle(w463) -> ("X"=w449:sgl, "Y"=w448:sgl, "Z"=w447:sgl)
                n230 = Unbundle(w462) -> ("X"=w446:sgl, "Y"=w445:sgl, "Z"=w444:sgl)
                n231 = formula code="float32 ux, uy, uz,vx, vy, vz; \nfloat32 cx,cy,cz; \nux = p1x - p0x; \nuy = p1y - p0y; \nuz = p1z - p0z; \nvx = p2x - p0x; \nvy = p2y - p0y; \nvz = p2z - p0z; \ncx = uy*vz - uz*vy;\ncy = -ux*vz + uz*vx;\ncz = ux*vy - uy*vx;\na = -1/ (sqrt(cx*cx + cy*cy + cz*cz));\n//a = 1;"("p0x"=w461, "p0y"=w460, "p0z"=w459, "p1x"=w458, "p1y"=w457, "p1z"=w456, "p2x"=w455, "p2y"=w454, "p2z"=w453) -> ("cx"=w470:sgl, "cy"=w469:sgl, "cz"=w468:sgl, "a"=w471:dbl)
                n232 = formula code="float32 n0x,n0y,n0z,n1x,n1y,n1z,n2x,n2y,n2z;\ncx = a * cx; \ncy = a * cy; \ncz = a * cz; \nn0x = p0x + cx; \nn0y = p0y + cy;\nn0z = p0z + cz;\nn1x = p1x + cx; \nn1y = p1y + cy;\nn1z = p1z + cz;\nn2x = p2x + cx; \nn2y = p2y + cy;\nn2z = p2z + cz;"("p0x"=w452, "p0y"=w451, "p0z"=w450, "p1x"=w449, "p1y"=w448, "p1z"=w447, "p2x"=w446, "p2y"=w445, "p2z"=w444, "cx"=w470, "cy"=w469, "cz"=w468, "a"=w471) -> ("n0x"=w480:sgl, "n0y"=w479:sgl, "n0z"=w478:sgl, "n1x"=w477:sgl, "n1y"=w476:sgl, "n1z"=w475:sgl, "n2x"=w474:sgl, "n2y"=w473:sgl, "n2z"=w472:sgl)
                n233 = Bundle(w480, w479, w478) -> (w443:cluster{sgl, sgl, sgl})  [unwired: 1 in]
                n234 = Bundle(w477, w476, w475) -> (w442:cluster{sgl, sgl, sgl})  [unwired: 1 in]
                n235 = Bundle(w474, w473, w472) -> (w441:cluster{sgl, sgl, sgl})  [unwired: 1 in]
                n236 = Replace Array Subset(array=w483, new element #1=w443, index #1=w481, new element #2=w442, new element #3=w441) -> (w482:cluster{"X":sgl, "Y":sgl, "Z":sgl}[])  [unwired: 2 in]
              }
            }
          }
        }
      }
    }
    frame "Triangle Fan" {
      n237 = Array Size(array=w490) -> (size(s)=w486:i32)
      n238 = Greater?(x=w486, y=2) -> (0:w487:bool)
      n239 = case shown="\"Per Vertex\"" w485 {
        tunnel: w490 -> [_ w499 w543]
        tunnel: [cluster{"X":sgl, "Y":sgl, "Z":sgl}[] [{"X"=0.0, "Y"=0.0, "Z"=-1.0}] w498 w542] -> w489
        tunnel: w487 -> [_ w497 w541]
        tunnel: w486 -> [_ w492 w538]
        frame "Overall", Default {
        }
        frame "Per Primitive" {
          n240 = Subtract(x=w492, y=2) -> (x-y=w493:i32)
          n241 = Initialize Array(cluster{"X":sgl, "Y":sgl, "Z":sgl} {"X"=0.0, "Y"=0.0, "Z"=0.0} ("element"), w493) -> (w495:cluster{"X":sgl, "Y":sgl, "Z":sgl}[])
          n242 = case shown="True" w497 {
            tunnel: w499 -> [_ w505]
            tunnel: w495 -> [_ w504]
            tunnel: [_ w503] -> w498
            tunnel: w492 -> [_ w502]
            frame False {
            }
            frame True {
              n243 = Subtract(x=w502, y=2) -> (x-y=w500:i32)
              n244 = for {
                N: w500 -> [_]
                tunnel: w505 -> [w511]
                shift-right: [w509] -> w503
                shift-left: w504 -> [w510]
                i -> [w508]
                n245 = Index Array(array=w511, index #2=w508) -> (element #1=w536:cluster{"X":sgl, "Y":sgl, "Z":sgl}, element #2=w535:cluster{"X":sgl, "Y":sgl, "Z":sgl}, element #3=w537:cluster{"X":sgl, "Y":sgl, "Z":sgl})  [unwired: 2 in]
                n246 = Subtract(x=w535, y=w536) -> (x-y=w533:cluster{"X":sgl, "Y":sgl, "Z":sgl})
                n247 = Subtract(x=w537, y=w535) -> (x-y=w534:cluster{"X":sgl, "Y":sgl, "Z":sgl})
                n248 = Unbundle(w533) -> ("X"=w531:sgl, "Y"=w530:sgl, "Z"=w529:sgl)
                n249 = Unbundle(w534) -> ("X"=w528:sgl, "Y"=w527:sgl, "Z"=w532:sgl)
                n250 = Multiply(x=w530, y=w532) -> (x*y=w526:sgl)
                n251 = Multiply(x=w529, y=w527) -> (x*y=w525:sgl)
                n252 = Multiply(x=w529, y=w528) -> (x*y=w523:sgl)
                n253 = Multiply(x=w531, y=w532) -> (x*y=w524:sgl)
                n254 = Multiply(x=w531, y=w527) -> (x*y=w521:sgl)
                n255 = Multiply(x=w530, y=w528) -> (x*y=w522:sgl)
                n256 = Subtract(x=w526, y=w525) -> (x-y=w518:sgl)
                n257 = Subtract(x=w523, y=w524) -> (x-y=w517:sgl)
                n258 = Subtract(x=w521, y=w522) -> (x-y=w516:sgl)
                n259 = Square(x=w518) -> (x^2=w506:sgl)
                n260 = Square(x=w517) -> (x^2=w507:sgl)
                n261 = Square(x=w516) -> (x^2=w520:sgl)
                n262 = Bundle(w518, w517, w516) -> (w515:cluster{sgl, sgl, sgl})  [unwired: 1 in]
                n263 = Compound Arithmetic op=ADD(w506, w507, w520) -> (w519:sgl)
                n264 = Square Root(x=w519) -> (sqrt(x)=w514:sgl)
                n265 = Negate(x=w514) -> (-x=w512:sgl)
                n266 = Divide(x=w515, y=w512) -> (x/y=w513:cluster{sgl, sgl, sgl})
                n267 = Replace Array Subset(array=w510, new element=w513, index=w508) -> (w509:cluster{"X":sgl, "Y":sgl, "Z":sgl}[])
              }
            }
          }
        }
        frame "Per Vertex" {
          n268 = Initialize Array(cluster{"X":sgl, "Y":sgl, "Z":sgl} {"X"=0.0, "Y"=0.0, "Z"=0.0} ("element"), w538) -> (w539:cluster{"X":sgl, "Y":sgl, "Z":sgl}[])
          n269 = case shown="True" w541 {
            tunnel: w543 -> [_ w549]
            tunnel: w539 -> [_ w548]
            tunnel: [_ w547] -> w542
            tunnel: w538 -> [_ w546]
            frame False {
            }
            frame True {
              n270 = Subtract(x=w546, y=2) -> (x-y=w544:i32)
              n271 = for {
                N: w544 -> [_]
                tunnel: w549 -> [w598]
                shift-right: [w596] -> w547
                shift-left: w548 -> [w597]
                i -> [w595]
                n272 = Increment(x=w595) -> (x+1=w581:i32)
                n273 = Increment(x=w595) -> (x+1=w580:i32)
                n274 = Index Array(array=w598, index #2=w581) -> (element #1=w577:cluster{"X":sgl, "Y":sgl, "Z":sgl}, element #2=w578:cluster{"X":sgl, "Y":sgl, "Z":sgl}, element #3=w576:cluster{"X":sgl, "Y":sgl, "Z":sgl})  [unwired: 2 in]
                n275 = Index Array(array=w597, index #1=0 ("index"), index #2=w580) -> (element #1=w575:cluster{"X":sgl, "Y":sgl, "Z":sgl}, element #2=w574:cluster{"X":sgl, "Y":sgl, "Z":sgl}, element #3=w573:cluster{"X":sgl, "Y":sgl, "Z":sgl})  [unwired: 1 in]
                n276 = Unbundle(w577) -> ("X"=w572:sgl, "Y"=w571:sgl, "Z"=w570:sgl)
                n277 = Unbundle(w578) -> ("X"=w569:sgl, "Y"=w568:sgl, "Z"=w567:sgl)
                n278 = Unbundle(w576) -> ("X"=w566:sgl, "Y"=w565:sgl, "Z"=w564:sgl)
                n279 = Unbundle(w575) -> ("X"=w563:sgl, "Y"=w562:sgl, "Z"=w561:sgl)
                n280 = Unbundle(w574) -> ("X"=w560:sgl, "Y"=w559:sgl, "Z"=w558:sgl)
                n281 = Unbundle(w573) -> ("X"=w557:sgl, "Y"=w556:sgl, "Z"=w555:sgl)
                n282 = formula code="float32 ux, uy, uz,vx, vy, vz; \nfloat32 cx,cy,cz; \nux = p1x - p0x; \nuy = p1y - p0y; \nuz = p1z - p0z; \nvx = p2x - p0x; \nvy = p2y - p0y; \nvz = p2z - p0z; \ncx = uy*vz - uz*vy;\ncy = -ux*vz + uz*vx;\ncz = ux*vy - uy*vx;\na = -1/ (sqrt(cx*cx + cy*cy + cz*cz));\n//a = 1;"("p0x"=w572, "p0y"=w571, "p0z"=w570, "p1x"=w569, "p1y"=w568, "p1z"=w567, "p2x"=w566, "p2y"=w565, "p2z"=w564) -> ("cx"=w584:sgl, "cy"=w583:sgl, "cz"=w582:sgl, "a"=w585:dbl)
                n283 = formula code="float32 n0x,n0y,n0z,n1x,n1y,n1z,n2x,n2y,n2z;\ncx = a * cx; \ncy = a * cy; \ncz = a * cz; \nn0x = p0x + cx; \nn0y = p0y + cy;\nn0z = p0z + cz;\nn1x = p1x + cx; \nn1y = p1y + cy;\nn1z = p1z + cz;\nn2x = p2x + cx; \nn2y = p2y + cy;\nn2z = p2z + cz;"("p0x"=w563, "p0y"=w562, "p0z"=w561, "p1x"=w560, "p1y"=w559, "p1z"=w558, "p2x"=w557, "p2y"=w556, "p2z"=w555, "cx"=w584, "cy"=w583, "cz"=w582, "a"=w585) -> ("n0x"=w594:sgl, "n0y"=w593:sgl, "n0z"=w592:sgl, "n1x"=w591:sgl, "n1y"=w590:sgl, "n1z"=w589:sgl, "n2x"=w588:sgl, "n2y"=w587:sgl, "n2z"=w586:sgl)
                n284 = Bundle(w594, w593, w592) -> (w554:cluster{sgl, sgl, sgl})  [unwired: 1 in]
                n285 = Bundle(w591, w590, w589) -> (w553:cluster{sgl, sgl, sgl})  [unwired: 1 in]
                n286 = Bundle(w588, w587, w586) -> (w552:cluster{sgl, sgl, sgl})  [unwired: 1 in]
                n287 = Increment(x=w595) -> (x+1=w550:i32)
                n288 = Replace Array Subset(array=w597, new element #1=w554, index #1=0 ("index"), new element #2=w553, index #2=w550, new element #3=w552) -> (w596:cluster{"X":sgl, "Y":sgl, "Z":sgl}[])  [unwired: 1 in]
              }
            }
          }
        }
      }
    }
  }
  "Normal Array" <- w2
